vi "Initialize_Characterization_Tests.vi"() -> (0 "date/time":string, 2 "error out":errorcluster, 3 "Refnum out":refnum<k34>)   [LabVIEW 2019]
uses:
  SiPM_Tests_Global_Var.vi
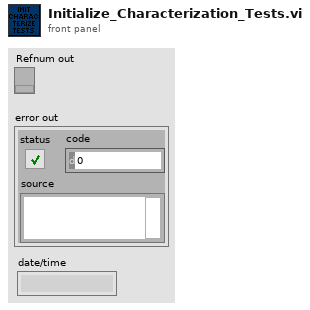
[diagram p1: front panel]
types:
  T1 = enum16{"big-endian, network order", "native, host order", "little-endian"}
  T2 = enum16{"open", "open or create", "create or replace", "create", "open (read-only)"}
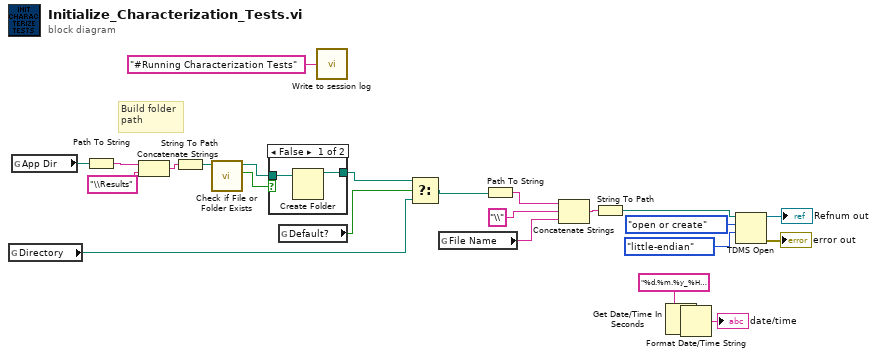
[diagram p0: block diagram]
diagram:
  # "Build folder\npath"
  n1 = global read "SiPM_Tests_Global_Var.vi" "Directory"() -> (w17:path)
  n2 = global read "SiPM_Tests_Global_Var.vi" "App Dir"() -> (w15:path)
  n3 = Path To String(path=w15) -> (string=w16:string)
  n4 = Concatenate Strings(w16, "\\Results" ("string")) -> (w14:string)
  n5 = String To Path(string=w14) -> (path=w13:path)
  n6 = call <vilib>:"Check if File or Folder Exists.vi"("path"=w13) -> ("file or folder exists?"=w12:bool, "dup path"=w11:path)  [unwired: 8 in, 1 out]
  n7 = case shown="False" w12 {
    tunnel: [w26 w27] -> w18
    tunnel: w11 -> [w25 w27]
    frame False {
      n8 = Create Folder(path (use dialog)=w25) -> (created path=w26:path)  [unwired: 2 in, 2 out]
    }
    frame True {
    }
  }
  n9 = global read "SiPM_Tests_Global_Var.vi" "Default?"() -> (w19:bool)
  n10 = call "Write to session log.vi"("Session string"="#Running Characterization Tests") -> ()  [unwired: 1 in]
  n11 = Select(t=w18, s=w19, f=w17) -> (s? t:f=w3:path)
  n12 = global read "SiPM_Tests_Global_Var.vi" "File Name"() -> (w2:string)
  n13 = Path To String(path=w3) -> (string=w5:string)
  n14 = Concatenate Strings(w5, "\\" ("string"), w2) -> (w4:string)
  n15 = String To Path(string=w4) -> (path=w1:path)
  n16 = Get Date/Time In Seconds() -> (seconds since 1Jan1904=w9:timestamp)
  n17 = Format Date/Time String(time format string (%c)="%d.%m.%y_%H.%M_", seconds (now)=w9) -> (date/time string=→"date/time":string)  [unwired: 1 in]
  n18 = TDMS Open(9:T1."little-endian" ("byte order (2:little-endian)"), 10:T2."open or create" ("operation (0:open)"), 11:w1) -> (0:→"error out":errorcluster, 3:→"Refnum out":refnum<k34>)  [unwired: 4 in]
